vi "clear Session Data.vi"(0 "Session in":refnum<class "Configurations.lvclass">=refnum, 11 "error in":errorcluster) -> (4 "Session out":refnum<class "Configurations.lvclass">, 15 "error out":errorcluster)   [LabVIEW 2016, in "_Configurations.lvlib" / "Configurations.lvclass"]
uses:
  Configurations.lvclass
  <vilib>/Utility/config.llb/NI_LVConfig.lvlib
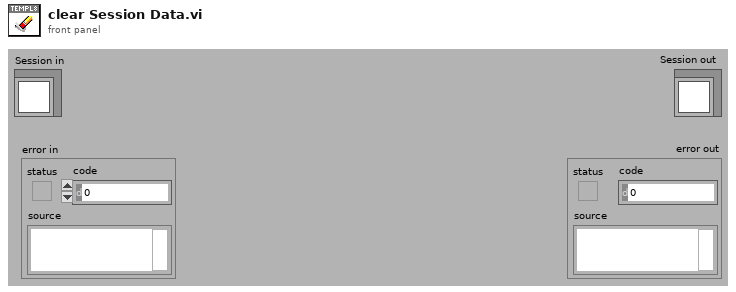
[diagram p1: front panel]
types:
  T1 = typedef "NI_LVConfig.lvlib/Config Data RefNum.ctl" = refnum<k1>
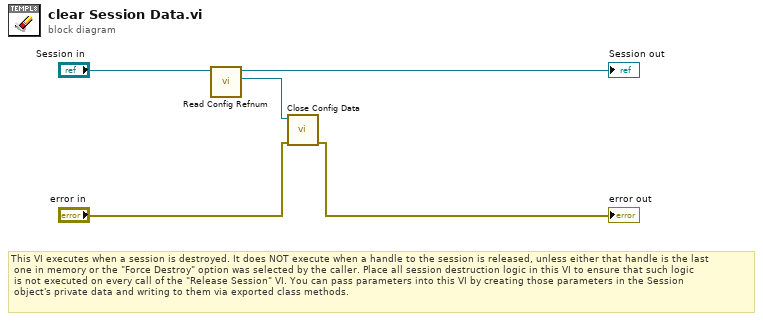
[diagram p0: block diagram]
diagram:
  # "This VI executes when a session is destroyed. It does NOT execute when a handle to the session is released, unless either that handle is the last\n one in memory or the \"Force Destroy\" option was selected by the caller. Place all session destruction logic in this VI to ensure that such logic\n is not executed on every call of the \"Release Session\" VI. You can pass parameters into this VI by creating those parameters in the Session \n object's private data and writing to them via exported class methods."
  n1 = call-dynamic "Read Config Refnum.vi"("Configurations in"="Session in") -> ("config data"=w3:T1, "Configurations out"=→"Session out":refnum<class "Configurations.lvclass">)  [unwired: 9 in]
  n2 = call <vilib>:"Close Config Data.vi"("error in (no error)"="error in", "refnum"=w3) -> ("error out"=→"error out":errorcluster)  [unwired: 8 in, 1 out]
